vi "Is slot empty.vi"(8 "error in (no error)":errorcluster, 10 "Card Position":T2={"Rack #"=0, "Slot #"=1} {"Slot #" max=15}, 11 "Devcie Ref in":T1 format="%.0x") -> (0 "error out":errorcluster, 1 "Empty?":bool, 3 "Device Ref out":T1 format="%.0x")   [LabVIEW 2014, in "SLSC configuration System Explorer.lvlib"]
uses:
  SLSC configuration System Explorer.lvlib
  Type Defs/Card Position.ctl
  Shared/SPI Utility/Slot #.ctl
  <vilib>/NI Veristand/Custom Device API/Custom Device Item Ref.ctl
  Shared/Constants.vi
  <vilib>/NI Veristand/Custom Device API/Get Item Property (U16).vi
  <vilib>/NI Veristand/Custom Device API/Custom Device API.lvlib
  Shared/SLSC configuration Shared.lvlib
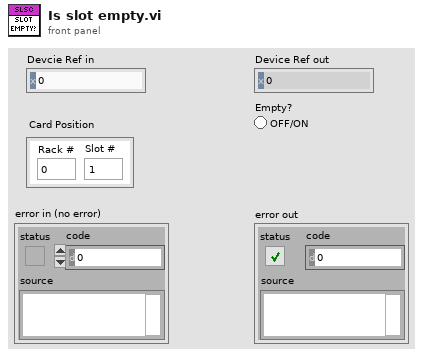
[diagram p1: front panel]
types:
  T1 = typedef "Custom Device API.lvlib/Custom Device Item Ref.ctl" = u64
  T2 = typedef "SLSC configuration Shared.lvlib/Card Position.ctl" = cluster{"Rack #":u8, "Slot #":T3}
  T3 = typedef "SLSC configuration Shared.lvlib/Slot #.ctl" = u8
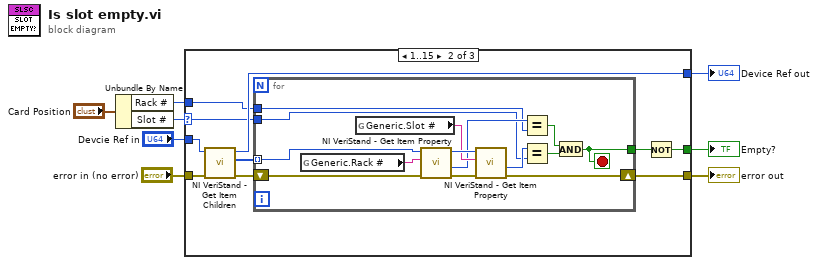
[diagram p0: block diagram]
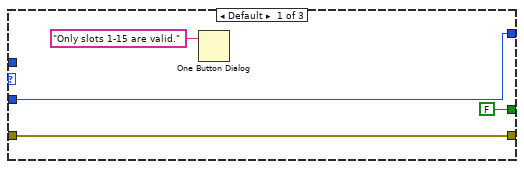
[diagram p2: hidden frame]
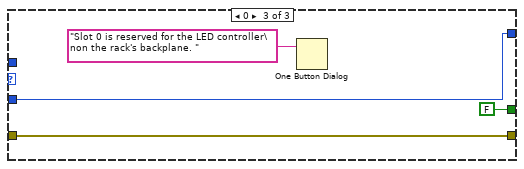
[diagram p3: hidden frame]
diagram:
  n1 = Unbundle By Name("Card Position") -> ("Rack #"=w3:u8, "Slot #"=w4:T3)
  n2 = case shown="1..15" w4 {
    selector: w4 -> [_ w13 _]
    tunnel: [FALSE w21 FALSE] -> w8
    tunnel: "error in (no error)" -> [w11 w20 w39]
    tunnel: [w11 w18 w39] -> w7
    tunnel: "Devcie Ref in" -> [w12 w16 w40]
    tunnel: [w12 w15 w40] -> w6
    tunnel: w3 -> [_ w14 _]
    frame Default {
      n3 = One Button Dialog(message="Only slots 1-15 are valid.") -> ()  [unwired: 1 in, 1 out]
    }
    frame 1..15 {
      n4 = call <vilib>:"NI VeriStand - Get Item Children.vi"("error in (no error)"=w20, "Item Ref in"=w16) -> ("error out"=w19:errorcluster, "Child Refs"=w17:T1[], "Item Ref out"=w15:T1)  [unwired: 6 in, 1 out]
      n5 = for {
        tunnel: [w25] -> w22
        shift-right: [w30] -> w18
        shift-left: w19 -> [w35]
        tunnel: w17 -> [w34] mode=indexing
        tunnel: w14 -> [w24]
        tunnel: w13 -> [w23]
        stop <- w25 stop-if-true
        n6 = global read "Constants.vi" "Generic.Rack #"() -> (w36:string)
        n7 = global read "Constants.vi" "Generic.Slot #"() -> (w31:string)
        n8 = call-poly <vilib>:"NI VeriStand - Get Item Property.vi"("error in (no error)"=w35, "Property Name"=w36, "Item Ref in"=w34) -> ("error out"=w33:errorcluster, "Value"=w29:u16, "Item Ref out"=w32:T1)  [unwired: 5 in, 1 out]
        n9 = call-poly <vilib>:"NI VeriStand - Get Item Property.vi"("error in (no error)"=w33, "Property Name"=w31, "Item Ref in"=w32) -> ("error out"=w30:errorcluster, "Value"=w28:u16)  [unwired: 5 in, 2 out]
        n10 = Equal?(x=w29, y=w24) -> (x = y?=w26:bool)
        n11 = Equal?(x=w28, y=w23) -> (x = y?=w27:bool)
        n12 = And(x=w26, y=w27) -> (x .and. y?=w25:bool)
      }
      n13 = Not(x=w22) -> (.not. x?=w21:bool)
    }
    frame 0 {
      n14 = One Button Dialog(message="Slot 0 is reserved for the LED controller\non the rack's backplane. ") -> ()  [unwired: 1 in, 1 out]
    }
  }
  "Empty?" <- w8
  "error out" <- w7
  "Device Ref out" <- w6
